vi "Write num of images.vi"(8 "error in (no error)":errorcluster, 10 "# of images":u32, 11 "Camera in":refnum<class "Camera.lvclass">) -> (0 "error out":errorcluster, 3 "Camera out":refnum<class "Camera.lvclass">)   [LabVIEW 2013, in "Camera.lvclass"]
uses:
  Camera.lvclass
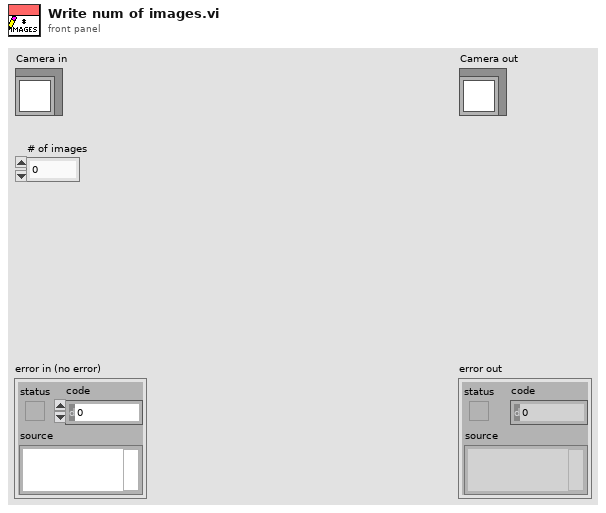
[diagram p1: front panel]
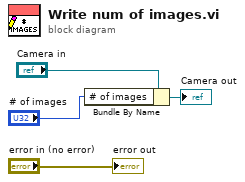
[diagram p0: block diagram]
diagram:
  n1 = Bundle By Name(cluster="Camera in", "# of images"="# of images") -> (→"Camera out":refnum<class "Camera.lvclass">)
  "error out" <- "error in (no error)"
